vi "data acquisition.vi"(1 "samples per acquisition":dbl, 2 "samples rate":dbl) -> ()   [LabVIEW 2014]
panel:
  in  "OK Button":bool
  out "Waveform Graph":dbl[](graph)
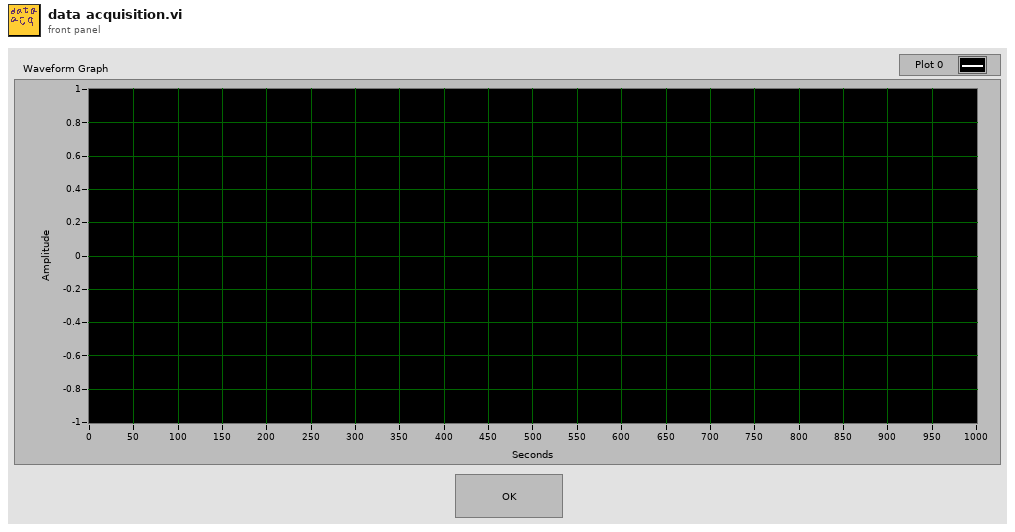
[diagram p1: front panel]
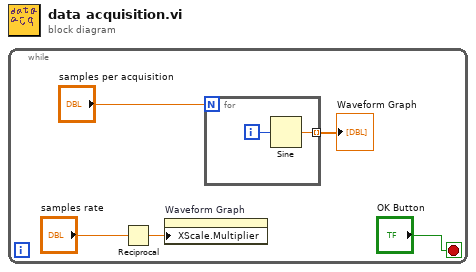
[diagram p0: block diagram]
diagram:
  n1 = while {
    stop <- "OK Button" stop-if-true
    n2 = Reciprocal(x="samples rate") -> (1/x=w3:dbl)
    n3 = property on="Waveform Graph" class="WFGraph (strict)"("XScale.Multiplier"=w3) -> ()  [unwired: 2 in, 2 out]
    n4 = for {
      N: "samples per acquisition" -> [_]
      tunnel: [w7] -> w5 mode=indexing
      i -> [w6]
      n5 = Sine(x=w6) -> (sin(x)=w7:dbl)
    }
    "Waveform Graph" <- w5
  }
